vi "gyro -- async pll engine V2 owl.vi"(11 "pll engine event pair":T11) -> ()   [LabVIEW 2021]
uses:
  PID action.ctl
  pll parameters.ctl
  PID - mode.ctl
  lorentzian.ctl
  circle corners.ctl
  pll talkback data type.ctl
  server talk-to-back pair.ctl
  server talkback message type.ctl
  server talkto message type.ctl
  pid -- parameters.ctl
  owl parameters.ctl
  owl action.ctl
  owl -- send for fit action.ctl
  agregator -- action.ctl
  interpolation state - real.ctl
  launch items list.ctl
  que event bag action.ctl
  data source action.ctl
  four-corner circle transformation.ctl
  publisher action.ctl
  cursor winow.ctl
  linear interpolation - real.vi
  Q -- check range -- i -- real.vi
  linear interpolation iiii- complex.vi
  array -- sort 2D array -- Complex.vi/05c44075-957c-bc42-b6fa-2799d0bc0485.vi
  Q - not nan -- real.vi
  <vilib>/Array/Sort 2D Array - Pop Stack.vi
  <vilib>/Array/Sort 2D Array - Push Stack.vi
  array -- sort 2D array -- Complex.vi/05c44075-957c-bc42-b6fa-2799d0bc0485.vi/269d4b3b-47f5-49e3-8884-44851e4dd9d5.vi
  array -- sort 2D array -- Complex.vi/05c44075-957c-bc42-b6fa-2799d0bc0485.vi/6d99389c-673d-4efb-bf33-19b32bcf4cf8.vi
panel:
  in  "main":enum32{"Page 1", "Page 2", "Page 3"}(tab)
  in  "pll parameters":T1={"PID mode"=enum."normal", "plot time (sec)"=0.6, "dt (sec)"=0.1, "viscous time (sec)"=0.5, "dt ave time (sec)"=0.5, "PLL limit (Hz)"=5000.0} {"PLL limit (Hz)" format="%#.2f"; "dt ave time (sec)" format="%#_10f"; "viscous time (sec)" format="%#_10f"; "dt (sec)" format="%#_10f"; "plot time (sec)" format="%#_10f"}
  in  "PID parameters :{}[];'":T3={"I (sec)"=0.004634123928756344, "P (sec)"=0.008980860327047186} {"P (sec)" scale=0.01..10.0 scale format="%#_2p"; "I (sec)" scale=0.01..10.0 scale format="%#_2p"}
  out "results":T4={"ω (Hz)"=6.93618449166945e-310, "G (Hz)"=0.9683990629933289, "V (V)"=1e-323+8e-323i, "overlimit ?"=FALSE, "running lorentzian out"={"A (VHz)"=0.009142510077437082, "ω (Hz)"=0.020119879746428596, "Γ (Hz)"=0.8109571797025381, "φ (rad)"=2.007511093178386, "Q"=0.02481003960506107, "Norm  Ampl"=nan, "z∞ (V)"=0.018500144394306906-0.0037766698823995634i, "4corners"={"z (-pi/2)"=0.023947397893225086+0.01120736437940613i, "z(inf)"=0.018500144394306906-0.0037766698823995634i, "z (pi/2)"=0.0334841786561126-0.009223923381317745i, "z center"=0.028715788274668842+0.0009917204990441924i, "z(0)"=0.03893143215503078+0.005760110880487949i, "radius"=0.011273727277179521}}, "static lorentzian out"={"A (VHz)"=6.817921124952451, "ω (Hz)"=-1.0311345636926572, "Γ (Hz)"=-1.0311345636926572, "φ (rad)"=-1.0311345636926572, "Q"=-1.0311345636926572, "Norm  Ampl"=-1.0311345636926572, "z∞ (V)"=-1.0311345636926572+0.0i, "4corners"={"z (-pi/2)"=-1.0311345636926572+0.5736824521422934i, "z(inf)"=-0.5200164984937075+1.0975277942502903i, "z (pi/2)"=-1.0311345636926572+0.5736824521422934i, "z center"=-0.5136528600391839+0.580046090596817i, "z(0)"=-0.5200164984937075+1.0975277942502903i, "radius"=-1.0311345636926572}}} {"static lorentzian out"."z∞ (V)" format="%#_4p"; "static lorentzian out"."Q" format="%#_4p"; "static lorentzian out"."φ (rad)" format="%#_3p"; "static lorentzian out"."Γ (Hz)" format="%#_5p"; "static lorentzian out"."ω (Hz)" format="%#_9p"; "static lorentzian out"."A (VHz)" format="%#_3p"; "running lorentzian out"."z∞ (V)" format="%#_4p"; "running lorentzian out"."Q" format="%#_4p"; "running lorentzian out"."φ (rad)" format="%#_3p"; "running lorentzian out"."Γ (Hz)" format="%#_5p"; "running lorentzian out"."ω (Hz)" format="%#_9p"; "running lorentzian out"."A (VHz)" format="%#_3p"; "V (V)" format="%#_5p"; "G (Hz)" format="%#_5p"; "ω (Hz)" format="%#_11p"}
  out "PLL is ON ?":bool
  in  "OWL parameters":T7={"T (sec)"=3.0, "owl?"=enum."focus", "A (rad)"=0.8, "refit ?"=enum."chill"} {"T (sec)" scale=1.0..20.0; "A (rad)" scale=0.1..1.57}
  in  "publish dt (sec)":dbl=0.1 format="%#_10f"
  in  "fitter dt (sec)":dbl=0.1 format="%#_10f"
  in  "Do reset frequency -- PID action":T10=enum."reset frequency"
  in  "Do reset frequency source":dbl=15.0 format="%#_10f"
  out "zi freq temporary":dbl=46378.93366130424 format="%#.2f"
  out "DO reset freq !":bool
  in  "lorentzian":T5={"A (VHz)"=0.009142510077437082, "ω (Hz)"=0.020119879746428596, "Γ (Hz)"=0.8109571797025381, "φ (rad)"=2.007511093178386, "Q"=0.02481003960506107, "Norm  Ampl"=nan, "z∞ (V)"=0.018500144394306906-0.0037766698823995634i, "4corners"={"z (-pi/2)"=0.023947397893225086+0.01120736437940613i, "z(inf)"=0.018500144394306906-0.0037766698823995634i, "z (pi/2)"=0.0334841786561126-0.009223923381317745i, "z center"=0.028715788274668842+0.0009917204990441924i, "z(0)"=0.03893143215503078+0.005760110880487949i, "radius"=0.011273727277179521}} {"z∞ (V)" format="%#_4p"; "Q" format="%#_4p"; "φ (rad)" format="%#_3p"; "Γ (Hz)" format="%#_5p"; "ω (Hz)" format="%#_9p"; "A (VHz)" format="%#_3p"}
  out "PLL loop Stoped?":bool=TRUE
  out "publish loop Stoped?":bool=TRUE
  out "fitter loop Stoped?":bool=TRUE
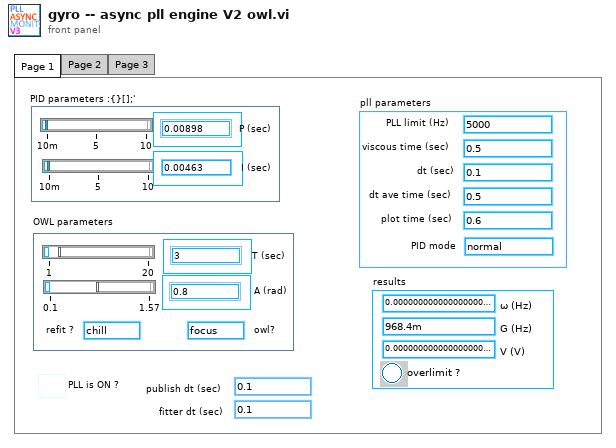
[diagram p1: front panel]
types:
  T1 = typedef "pll parameters.ctl" = cluster{"PID mode":T2, "plot time (sec)":dbl, "dt (sec)":dbl, "viscous time (sec)":dbl, "dt ave time (sec)":dbl, "PLL limit (Hz)":dbl}
  T2 = typedef "PID - mode.ctl" = enum16{"normal", "heat"}
  T3 = typedef "pid -- parameters.ctl" = cluster{"I (sec)":dbl, "P (sec)":dbl}
  T4 = typedef "pll talkback data type.ctl" = cluster{"ω (Hz)":dbl, "G (Hz)":dbl, "V (V)":cdb, "overlimit ?":bool, "running lorentzian out":T5, "static lorentzian out":T5}
  T5 = typedef "lorentzian.ctl" = cluster{"A (VHz)":dbl, "ω (Hz)":dbl, "Γ (Hz)":dbl, "φ (rad)":dbl, "Q":dbl, "Norm  Ampl":dbl, "z∞ (V)":cdb, "4corners":T6}
  T6 = typedef "circle corners.ctl" = cluster{"z (-pi/2)":cdb, "z(inf)":cdb, "z (pi/2)":cdb, "z center":cdb, "z(0)":cdb, "radius":dbl}
  T7 = typedef "owl parameters.ctl" = cluster{"T (sec)":dbl, "owl?":T8, "A (rad)":dbl, "refit ?":T9}
  T8 = typedef "owl action.ctl" = enum16{"owl", "focus"}
  T9 = typedef "owl -- send for fit action.ctl" = enum16{"refit", "chill"}
  T10 = typedef "PID action.ctl" = enum16{"append", "empty!", "reset frequency", "reset from num", "overlimit"}
  T11 = typedef "server talk-to-back pair.ctl" = cluster{"talkback event":refnum<user-event>, "talkto event":refnum<user-event>}
  T12 = typedef "launch items list.ctl" = enum16{"source", "pll engine", "pll monitor", "sweeper engine", "sweeper monitor", "fitter"}
  T13 = typedef "que event bag action.ctl" = enum16{"check", "add", "init", "keys", "values"}
  T14 = typedef "interpolation state - real.ctl" = cluster{"Array ":dbl[], "actual size":i32, "requested size":i32}
  T15 = typedef "agregator -- action.ctl" = enum16{"append", "interpolate", "empty!", "force", "init", "scale", "read last"}
  T16 = typedef "publisher action.ctl" = enum16{"set", "get", "init", "check"}
  T17 = typedef "server talkto message type.ctl" = cluster{"message":enum16{"stop", "start", "update pars", "update request", "new", "launch", "exit", "get", "reset", "pause", "unpause"}}
  T18 = typedef "data source action.ctl" = enum16{"set", "get", "init", "set-and-get", "init source"}
  T19 = typedef "four-corner circle transformation.ctl" = enum16{"z(c) z(inf)", "z(c) z(zero)", "fix phase", "calculate lorentzian", "z(0) z(+-pi/2)", "shift to zcenter", "to  canonical", "get canonical phase", "get4corners", "update lorentzian -- from z0", "fake gamma normal", "fake gamma heat", "calculate complex slope", "get f0 given f and phi"}
  T20 = typedef "cursor winow.ctl" = cluster{"left":dbl, "right ":dbl, "center":dbl, "window":dbl, "cursors":i32[], "relative":i32, "absolute":i32, "fixed vertical offset":dbl, "vertical offset":dbl, "skew":dbl, "default window frac":dbl, "kind":enum16{"symmetric", "skewed", "fancy"}, "skew.left":dbl, "skew.right":dbl, "Plot ref":refnum<vi>, "wing order":enum16{"forw", "back"}}
  T21 = typedef "PLL data source.ctl" = enum16{"meta", "MFLI", "SRS865A", "arydh"}
  T22 = typedef "interpolation state - complex.ctl" = cluster{"requested size":i32, "Array":cdb[], "actual number of elements":i32}
  T23 = typedef "server talkback message type.ctl" = cluster{"message":enum16{"new", "void"}}
  T24 = typedef "eventvkey.ctl" = enum16{"ASCII", "Enter", "Return", "Shift", "Ctrl", "Alt", "Cmd", "Opt", "Caps", "NumLock", "Clear", "Break", "Up", "Down", "Left", "Right", "Insert", "Delete", "Home", "End", "PageUp", "PageDown", "Escape", "Help", "Pause", "ScrollLock", "F1", "F2", "F3", "F4", "F5", "F6", "F7", "F8", "F9", "F10", "F11", "F12", "F13", "F14", "F15", "F16", "F17", "F18", "F19", "F20", "F21", "F22", "F23", "F24", "Play", "VolumeUp", "VolumeDown", "Mute", "Two Byte Char"}
  T25 = enum16{"stop", "start", "update pars", "update request", "new", "launch", "exit", "get", "reset", "pause", "unpause"}
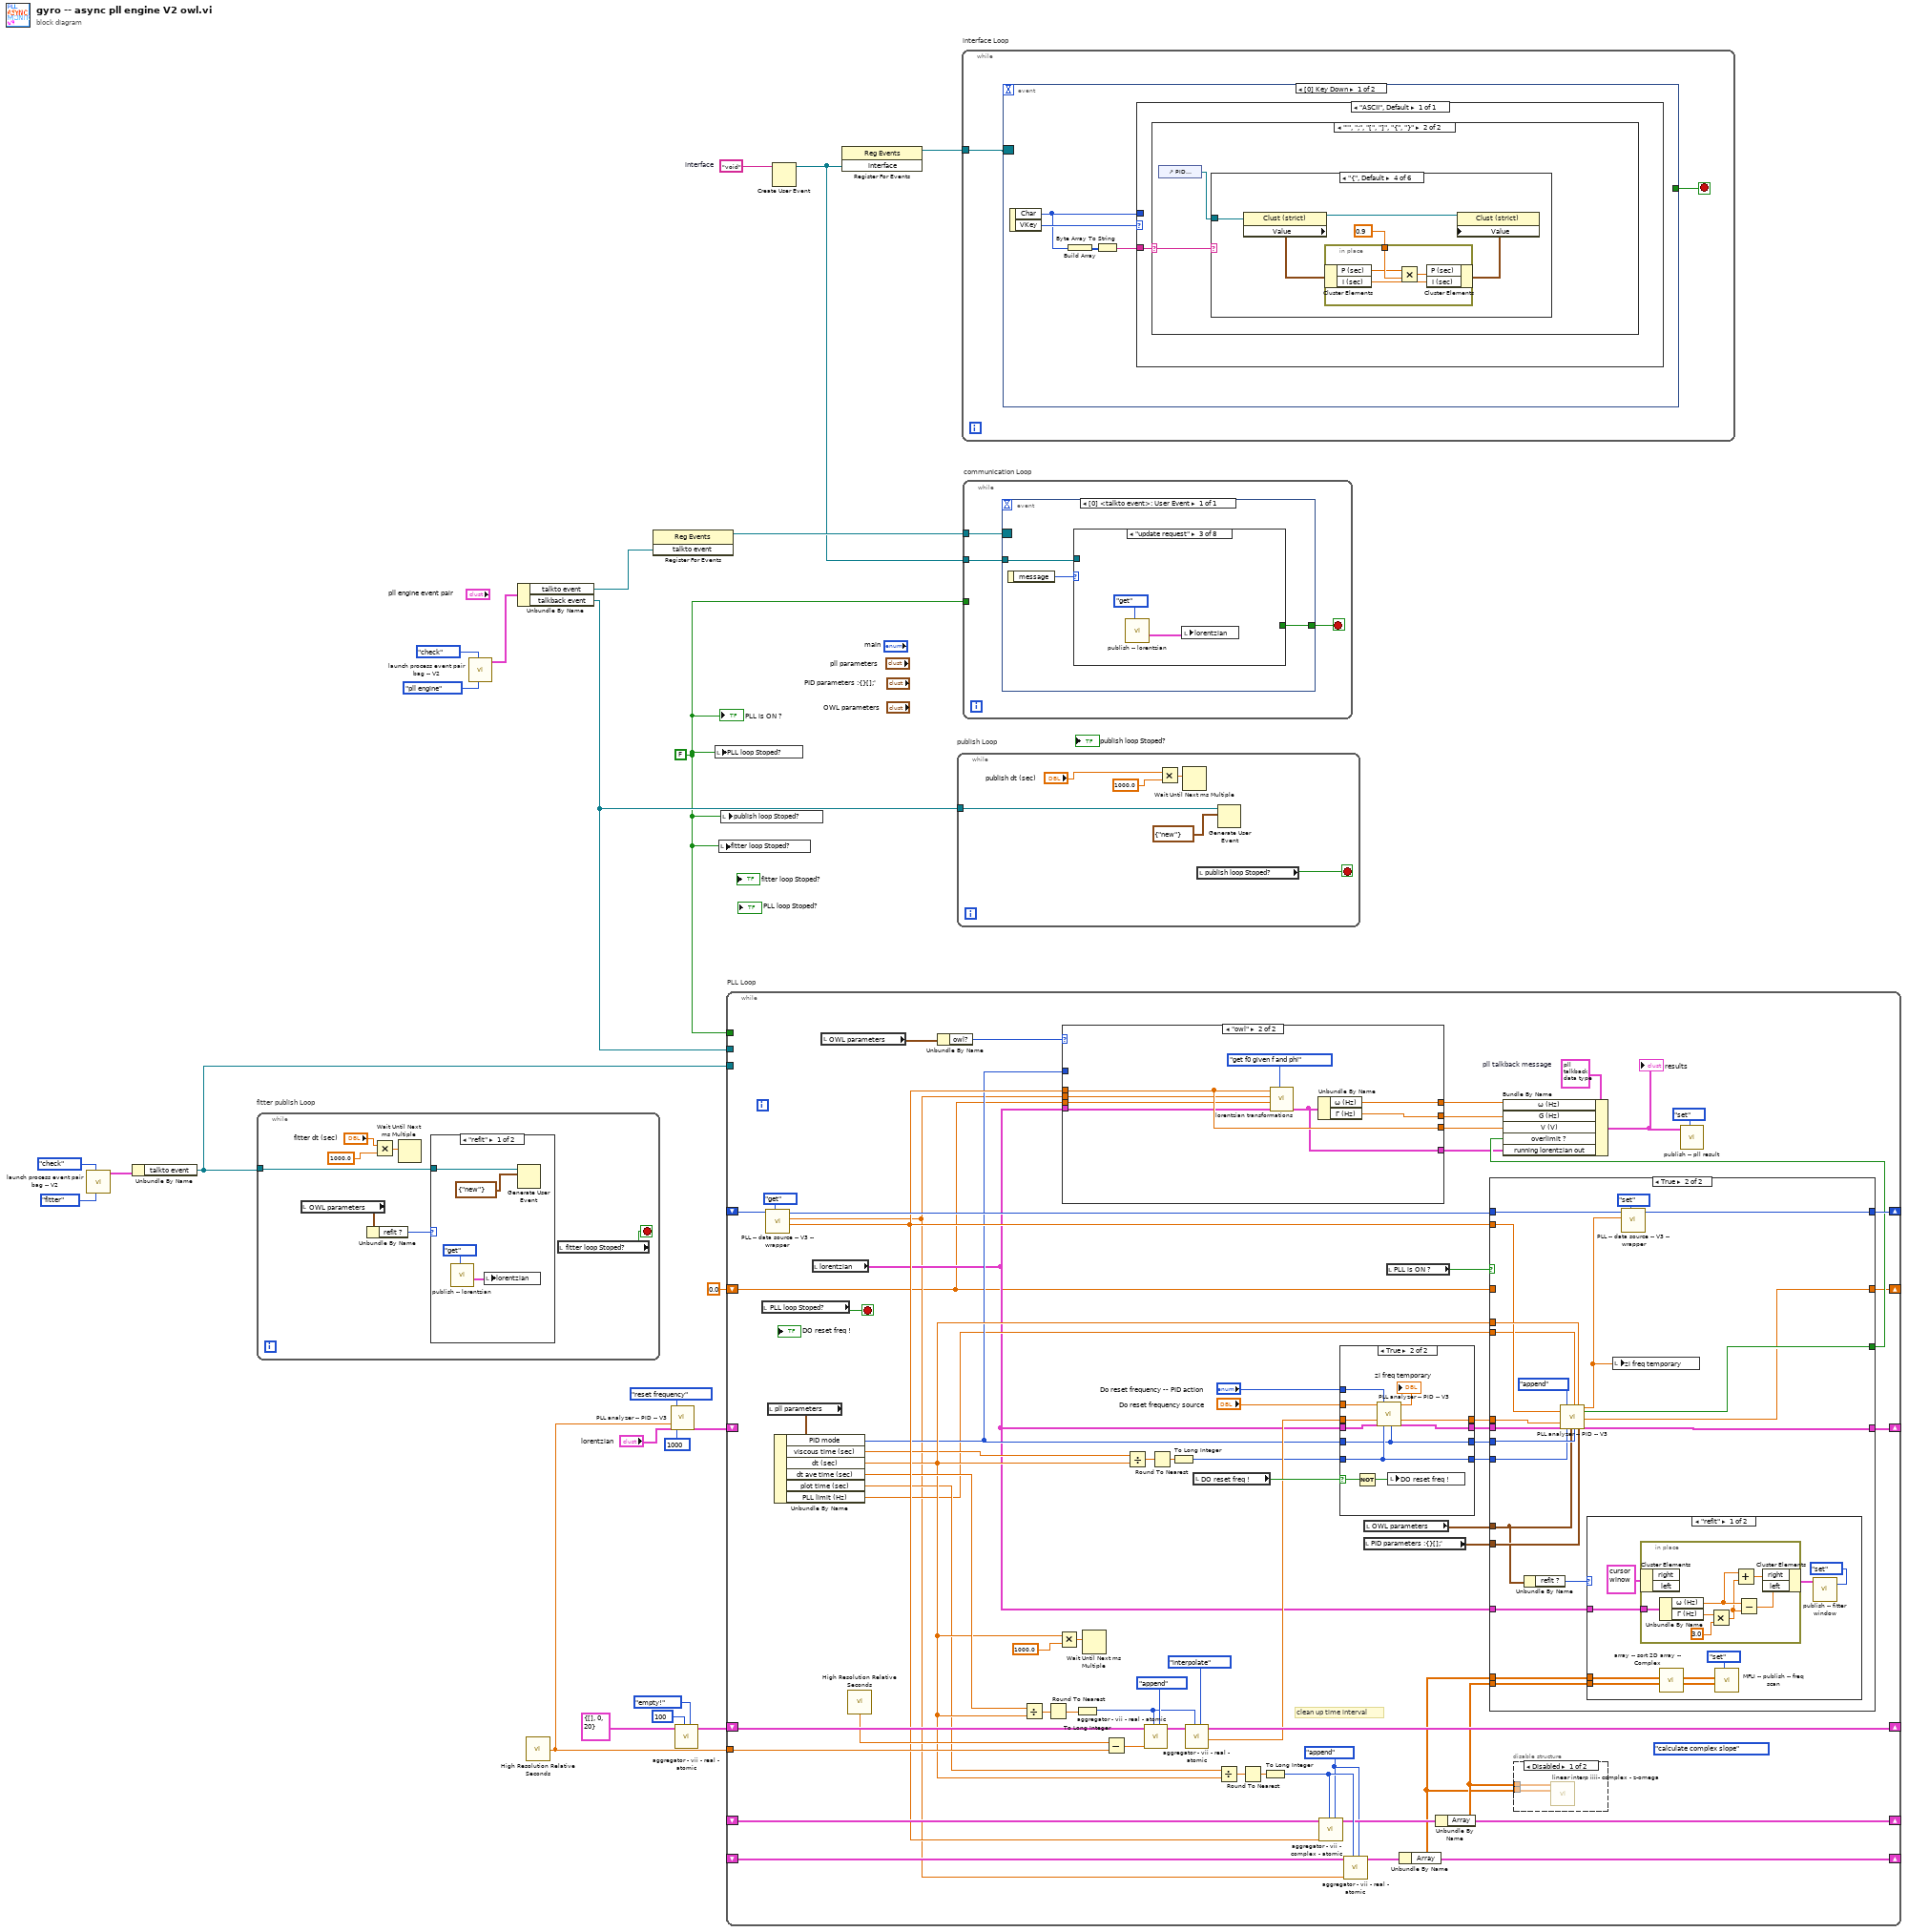
[diagram p0: block diagram]
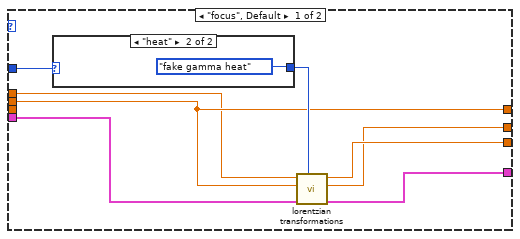
[diagram p3: hidden frame]
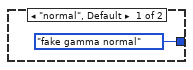
[diagram p4: hidden frame]
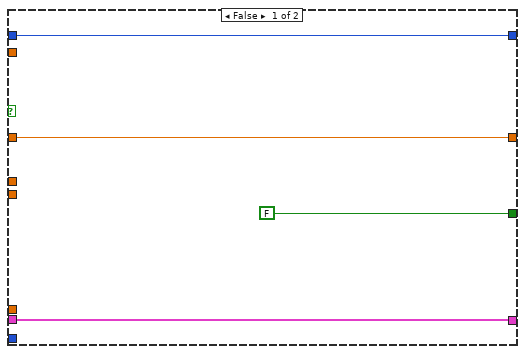
[diagram p6: hidden frame]
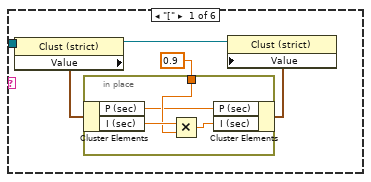
[diagram p10: hidden frame]
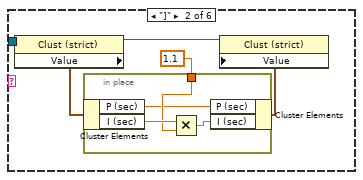
[diagram p11: hidden frame]
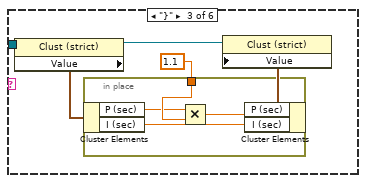
[diagram p12: hidden frame]
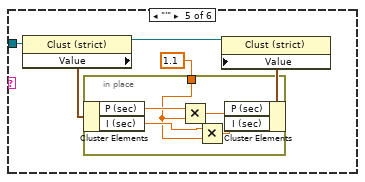
[diagram p13: hidden frame]
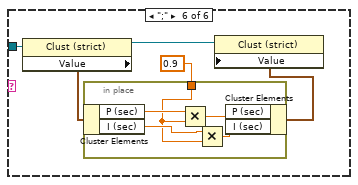
[diagram p14: hidden frame]
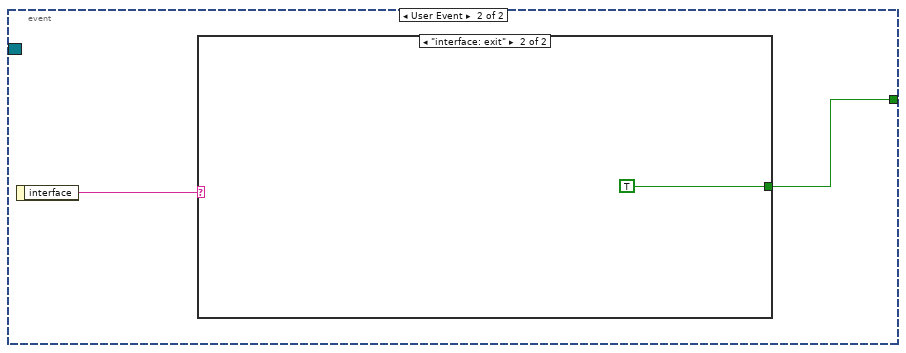
[diagram p15: hidden frame]
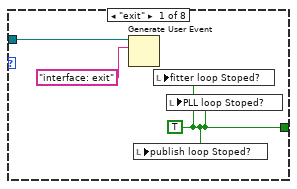
[diagram p17: hidden frame]
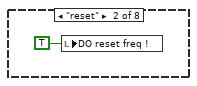
[diagram p18: hidden frame]
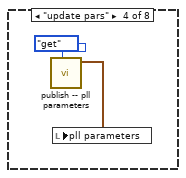
[diagram p19: hidden frame]
diagram:
  w13 = "void"  # interface
  w3 = FALSE ("Stop")
  n1 = call "launch process event pair bag -- V2.vi"("launch item"=launch_items_list."fitter" ("launch items"), "bag action"=que_event_bag_action."check") -> ("event pair OUT"=w4:T11)  [unwired: 7 in, 2 out]
  n2 = Unbundle By Name(w4) -> ("talkto event"=w2:refnum<user-event>)
  n3 = while "fitter publish Loop" {
    tunnel: w2 -> [w31]
    stop <- w30 stop-if-true
    n4 = local read "OWL parameters"() -> (w26:T7)
    n5 = Unbundle By Name(w26) -> ("refit ?"=w25:T9)
    n6 = Multiply(x="fitter dt (sec)", y=1000.0) -> (x*y=w27:dbl)
    n7 = Wait Until Next ms Multiple(millisecond multiple=w27) -> ()  [unwired: 1 out]
    n8 = case shown="\"refit\"" w25 {
      tunnel: w31 -> [w35 _]
      frame "refit" {
        n9 = call "publish -- lorentzian.vi"("publisher action"=publisher_action."get") -> ("lorentzian OUT"=w32:T5)  [unwired: 10 in]
        n10 = local write "lorentzian"(w32) -> ()
        n11 = Generate User Event(user event=w35, event data cluster=T17 {"message"=enum."new"} ("event data")) -> ()  [unwired: 2 in, 2 out]
      }
      frame "chill", Default {
      }
    }
    n12 = local read "fitter loop Stoped?"() -> (w30:bool)
  }
  n13 = call "launch process event pair bag -- V2.vi"("launch item"=launch_items_list."pll engine" ("launch items"), "bag action"=que_event_bag_action."check") -> ("event pair OUT"=w7:T11)  [unwired: 7 in, 2 out]
  n14 = Unbundle By Name(w7) -> ("talkto event"=w23:refnum<user-event>, "talkback event"=w10:refnum<user-event>)
  n15 = call <vilib>:"High Resolution Relative Seconds.vi"() -> ("relative seconds"=w15:dbl)
  n16 = register-events(w23) -> (reference out=w24:refnum<event-registration>)  [unwired: 2 in, 1 out]
  n17 = call "PLL analyzer -- PID -- V3.vi"("time in (sec)"=w15, "lorentzian IN"="lorentzian", "PID action"=PID_action."reset frequency", "requested size"=1000) -> ("lorentzian  OUT"=w18:T5)  [unwired: 11 in, 4 out]
  n18 = call "aggregator - vii - real - atomic.vi"("aggregator action"=agregator_--_action."empty!", "requested size"=100, "state IN"=T14 {"Array "=[], "actual size"=0, "requested size"=20}) -> ("state OUT"=w21:T14)  [unwired: 5 in, 3 out]
  n19 = local write "PLL loop Stoped?"(w3) -> ()
  n20 = local write "fitter loop Stoped?"(w3) -> ()
  n21 = local write "publish loop Stoped?"(w3) -> ()
  n22 = while "PLL Loop" {
    tunnel: w15 -> [w100]
    shift-right: [w98] -> _
    shift-left: w18 -> [_]
    shift-right: [w66] -> _
    shift-left: _ -> [w97]
    shift-right: [w95] -> _
    shift-left: _ -> [w96]
    shift-right: [w90] -> _
    shift-left: w21 -> [w93]
    shift-right: [w85] -> _
    shift-left: _ -> [w81]
    tunnel: w10 -> [_]
    tunnel: w3 -> [_]
    tunnel: w2 -> [_]
    shift-right: [w37] -> _
    shift-left: 0.0 ("phase OUT (rad)") -> [w36]
    stop <- w51 stop-if-true
    w62 = T4 {"ω (Hz)"=0.0, "G (Hz)"=0.0, "V (V)"=0.0+0.0i, "overlimit ?"=FALSE, "running lorentzian out"={"A (VHz)"=-1.0311345636926572, "ω (Hz)"=-1.0311345636926572, "Γ (Hz)"=-1.0311345636926572, "φ (rad)"=-1.0311345636926572, "Q"=-1.0311345636926572, "Norm  Ampl"=-1.0311345636926572, "z∞ (V)"=-1.0311345636926572+0.0i, "4corners"={"z (-pi/2)"=-1.0311345636926572+0.5736824521422934i, "z(inf)"=-0.5200164984937075+1.0975277942502903i, "z (pi/2)"=-1.0311345636926572+0.5736824521422934i, "z center"=-0.5136528600391839+0.580046090596817i, "z(0)"=-0.5200164984937075+1.0975277942502903i, "radius"=-1.0311345636926572}}, "static lorentzian out"={"A (VHz)"=6.817921124952451, "ω (Hz)"=-1.0311345636926572, "Γ (Hz)"=-1.0311345636926572, "φ (rad)"=-1.0311345636926572, "Q"=-1.0311345636926572, "Norm  Ampl"=-1.0311345636926572, "z∞ (V)"=-1.0311345636926572+0.0i, "4corners"={"z (-pi/2)"=-1.0311345636926572+0.5736824521422934i, "z(inf)"=-0.5200164984937075+1.0975277942502903i, "z (pi/2)"=-1.0311345636926572+0.5736824521422934i, "z center"=-0.5136528600391839+0.580046090596817i, "z(0)"=-0.5200164984937075+1.0975277942502903i, "radius"=-1.0311345636926572}}}  # pll talkback message
    (unwired) four-corner_circle_transformation."calculate complex slope" ("4 corner circle transformation")
    w48 = agregator_--_action."append" ("aggregator action")
    # "clean up time interval"
    n23 = local read "PLL loop Stoped?"() -> (w51:bool)
    n24 = call "PLL -- data source -- V3 -- wrapper.vi"("data source action"=data_source_action."get", "PLL data source"=w81) -> ("z out (V)"=w63:cdb, "Freq out (Hz)"=w43:dbl, "PLL data source OUT"=w83:T21)  [unwired: 7 in]
    n25 = local read "pll parameters"() -> (w57:T1)
    n26 = Unbundle By Name(w57) -> ("PID mode"=w58:T2, "viscous time (sec)"=w59:dbl, "dt (sec)"=w60:dbl, "dt ave time (sec)"=w61:dbl, "plot time (sec)"=w56:dbl, "PLL limit (Hz)"=w54:dbl)
    n27 = local read "lorentzian"() -> (w44:T5)
    n28 = local read "OWL parameters"() -> (w39:T7)
    n29 = call <vilib>:"High Resolution Relative Seconds.vi"() -> ("relative seconds"=w84:dbl)
    n30 = Unbundle By Name(w39) -> ("owl?"=w40:T8)
    n31 = Divide(x=w61, y=w60) -> (x/y=w74:dbl)
    n32 = Round To Nearest(number=w74) -> (nearest integer value=w73:dbl)
    n33 = Multiply(x=w60, y=1000.0) -> (x*y=w88:dbl)
    n34 = case shown="\"owl\"" w40 {
      tunnel: [w101 w114] -> w64
      tunnel: w63 -> [w103 w116]
      tunnel: w58 -> [w105 _]
      tunnel: w44 -> [w102 w112]
      tunnel: w43 -> [w104 w113]
      tunnel: [w104 w111] -> w42
      tunnel: [w103 w116] -> w41
      tunnel: [w102 w110] -> w38
      tunnel: w36 -> [_ w109]
      frame "focus", Default {
        n35 = case shown="\"heat\"" w105 {
          tunnel: [four-corner_circle_transformation."fake gamma normal" ("4 corner circle transformation") four-corner_circle_transformation."fake gamma heat" ("4 corner circle transformation")] -> w106
          frame "normal", Default {
          }
          frame "heat" {
          }
        }
        n36 = call "lorentzian transformations.vi"("4 corner circle transformation"=w106, "lorentzian in"=w102, "freq in"=w104, "voltage in"=w103) -> ("gamma OUT"=w101:dbl)  [unwired: 4 in, 3 out]
      }
      frame "owl" {
        n37 = call "lorentzian transformations.vi"("4 corner circle transformation"=four-corner_circle_transformation."get f0 given f and phi", "lorentzian in"=w112, "phase in (rad)"=w109, "freq in"=w113, "voltage in"=w116) -> ("lorentzian out"=w110:T5)  [unwired: 3 in, 3 out]
        n38 = Unbundle By Name(w110) -> ("ω (Hz)"=w111:dbl, "Γ (Hz)"=w114:dbl)
      }
    }
    n39 = To Long Integer(number=w73) -> (32bit integer=w72:i32)
    n40 = Wait Until Next ms Multiple(millisecond multiple=w88) -> ()  [unwired: 1 out]
    n41 = Subtract(x=w84, y=w100) -> (x-y=w92:dbl)
    n42 = Divide(x=w59, y=w60) -> (x/y=w77:dbl)
    n43 = call "aggregator - vii - real - atomic.vi"("aggregator action"=agregator_--_action."append", "requested size"=w72, "number"=w92, "state IN"=w93) -> ("state OUT"=w91:T14)  [unwired: 4 in, 3 out]
    n44 = Round To Nearest(number=w77) -> (nearest integer value=w76:dbl)
    n45 = To Long Integer(number=w76) -> (32bit integer=w75:i32)
    n46 = call "aggregator - vii - real - atomic.vi"("aggregator action"=agregator_--_action."interpolate", "requested size"=w72, "state IN"=w91) -> ("interp average"=w79:dbl, "state OUT"=w90:T14)  [unwired: 5 in, 2 out]
    n47 = local read "DO reset freq !"() -> (w87:bool)
    n48 = Divide(x=w56, y=w60) -> (x/y=w70:dbl)
    n49 = Round To Nearest(number=w70) -> (nearest integer value=w69:dbl)
    n50 = To Long Integer(number=w69) -> (32bit integer=w68:i32)
    n51 = call "aggregator - vii - complex - atomic.vi"("aggregator action"=w48, "requested size"=w68, "number"=w63, "state IN"=w97) -> ("state OUT"=w66:T22)  [unwired: 4 in, 3 out]
    n52 = case shown="True" w87 {
      selector: w87 -> [_ w172]
      tunnel: w44 -> [w163 w174]
      tunnel: [w163 w173] -> w86
      tunnel: w75 -> [w162 w169]
      tunnel: [w162 w169] -> w80
      tunnel: w79 -> [w161 w168]
      tunnel: "Do reset frequency -- PID action" -> [_ w167]
      tunnel: "Do reset frequency source" -> [_ w166]
      tunnel: [w161 w165] -> w71
      tunnel: w58 -> [w160 w164]
      tunnel: [w160 w164] -> w67
      frame False {
      }
      frame True {
        n53 = Not(x=w172) -> (.not. x?=w171:bool)
        n54 = call "PLL analyzer -- PID -- V3.vi"("frequency IN (Hz)"=w166, "time in (sec)"=w168, "lorentzian IN"=w174, "PID action"=w167, "requested size"=w169, "PID mode"=w164) -> ("frequency OUT (Hz)"=→"zi freq temporary":dbl, "time out (sec)"=w165:dbl, "lorentzian  OUT"=w173:T5)  [unwired: 9 in, 2 out]
        n55 = local write "DO reset freq !"(w171) -> ()
      }
    }
    n56 = call "aggregator - vii - real - atomic.vi"("aggregator action"=w48, "requested size"=w68, "number"=w43, "state IN"=w96) -> ("state OUT"=w95:T14)  [unwired: 4 in, 3 out]
    n57 = local read "PID parameters :{}[];'"() -> (w49:T3)
    n58 = local read "OWL parameters"() -> (w47:T7)
    n59 = local read "PLL is ON ?"() -> (w50:bool)
    n60 = Unbundle By Name(w95) -> ("Array"=w45:dbl[])
    n61 = Unbundle By Name(w66) -> ("Array"=w46:cdb[])
    n62 = case shown="True" w50 {
      tunnel: [w122 w143] -> w98
      tunnel: w80 -> [_ w134]
      tunnel: w63 -> [_ w133]
      tunnel: w71 -> [_ w138]
      tunnel: w86 -> [w122 w135]
      tunnel: [w121 w141] -> w85
      tunnel: w83 -> [w121 w139]
      tunnel: w60 -> [_ w137]
      tunnel: w67 -> [_ w136]
      tunnel: w49 -> [_ w132]
      tunnel: [FALSE w131] -> w55
      tunnel: w54 -> [_ w130]
      tunnel: w47 -> [_ w127]
      tunnel: w46 -> [_ w129]
      tunnel: w45 -> [_ w128]
      tunnel: w44 -> [_ w125]
      tunnel: [w119 w123] -> w37
      tunnel: w36 -> [w119 _]
      frame False {
      }
      frame True {
        n63 = Unbundle By Name(w127) -> ("refit ?"=w126:T9)
        n64 = call "PLL analyzer -- PID -- V3.vi"("voltage IN (V)"=w133, "time in (sec)"=w138, "lorentzian IN"=w135, "PID action"=PID_action."append", "requested size"=w134, "OWL parameters"=w127, "PLL limits (Hz)"=w130, "PID mode"=w136, "dt (sec)"=w137, "PID parameters"=w132) -> ("frequency OUT (Hz)"=w124:dbl, "overlimit ?"=w131:bool, "phase OUT (rad)"=w123:dbl, "lorentzian  OUT"=w143:T5)  [unwired: 5 in, 1 out]
        n65 = case shown="\"refit\"" w126 {
          tunnel: w129 -> [w145 _]
          tunnel: w128 -> [w147 _]
          tunnel: w125 -> [w149 _]
          frame "refit" {
            n66 = in-place {
              in-place-border: w149 -> [w159]
              n67 = in-place-cluster #1(T20 {"left"=-0.35260838541595674, "right "=17.234446484426172, "center"=-8.969831627629043, "window"=8.26461485679713, "cursors"=[], "relative"=0, "absolute"=0, "fixed vertical offset"=2421.6740576496672, "vertical offset"=2421.6740576496672, "skew"=2421.6740576496672, "default window frac"=2421.6740576496672, "kind"=enum."skewed", "skew.left"=2421.6740576496672, "skew.right"=2421.6740576496672, "Plot ref"=refnum, "wing order"=enum."back"} ("win OUT")) -> ()  [unwired: 2 out]
              n68 = Unbundle By Name(w159) -> ("ω (Hz)"=w156:dbl, "Γ (Hz)"=w158:dbl)
              n69 = Multiply(x=w158, y=3.0) -> (x*y=w155:dbl)
              n70 = Add(x=w156, y=w155) -> (x+y=w154:dbl)
              n71 = Subtract(x=w156, y=w155) -> (x-y=w153:dbl)
              n72 = in-place-cluster #1("right"=w154, "left"=w153) -> (w150:T20)
            }
            n73 = call "array -- sort 2D array -- Complex.vi"("z In"=w145, "freq IN"=w147) -> ("z out"=w144:cdb[], "freq out"=w146:dbl[])  [unwired: 8 in]
            n74 = call "MFLI -- publish -- freq scan.vi"("publisher action"=publisher_action."set", "Voltage IN (V)"=w144, "Freq IN (Hz)"=w146) -> ()  [unwired: 7 in, 2 out]
            n75 = call "publish -- fitter window.vi"("publisher action"=publisher_action."set", "win IN"=w150) -> ()  [unwired: 9 in, 1 out]
          }
          frame "chill", Default {
          }
        }
        n76 = local write "zi freq temporary"(w124) -> ()
        n77 = call "PLL -- data source -- V3 -- wrapper.vi"("data source action"=data_source_action."set", "Freq in (Hz)"=w124, "PLL data source"=w139) -> ("PLL data source OUT"=w141:T21)  [unwired: 6 in, 2 out]
      }
    }
    n78 = Bundle By Name(cluster=w62, "ω (Hz)"=w42, "G (Hz)"=w64, "V (V)"=w41, "overlimit ?"=w55, "running lorentzian out"=w38) -> (w53:T4)
    "results" <- w53
    n79 = disable-structure shown="Disabled" {
      disable-tunnel: w46 -> [w118 _]
      disable-tunnel: w45 -> [w117 _]
      frame Disabled {
        n80 = call "linear interp iiii- complex - z-omega.vi"("z"=w118, "omega"=w117) -> ()  [unwired: 5 in, 9 out]
      }
      frame Enabled {
      }
    }
    n81 = call "publish -- pll result.vi"("publisher action"=publisher_action."set", "pll result IN"=w53) -> ()  [unwired: 9 in, 1 out]
  }
  n82 = Create User Event(user event datatype=w13) -> (user event=w11:refnum<user-event>)  [unwired: 1 in, 1 out]
  n83 = register-events(w11) -> (reference out=w12:refnum<event-registration>)  [unwired: 2 in, 1 out]
  n84 = while "publish Loop" {
    tunnel: w10 -> [w179]
    stop <- w178 stop-if-true
    n85 = Multiply(x="publish dt (sec)", y=1000.0) -> (x*y=w175:dbl)
    n86 = Wait Until Next ms Multiple(millisecond multiple=w175) -> ()  [unwired: 1 out]
    n87 = local read "publish loop Stoped?"() -> (w178:bool)
    n88 = Generate User Event(user event=w179, event data cluster=T23 {"message"=enum."new"} ("event data")) -> ()  [unwired: 2 in, 2 out]
  }
  n89 = while "interface Loop" {
    tunnel: w12 -> [w182]
    stop <- w181 stop-if-true
    n90 = event shown="[0] Key Down" {
      selector: w182 -> [_ _]
      dyn-events: _ -> [_ _]
      timeout: _ -> [_ _]
      tunnel: [_ w246] -> w181
      event Key Down {
        n91 = event-data() -> ("Char"=w184:i16, "VKey"=w186:T24)  [unwired: 1 in]
        n92 = Build Array(w184) -> (w185:i16[])
        n93 = Byte Array To String(unsigned byte array=w185) -> (string=w183:string)
        n94 = case shown="\"ASCII\", Default" w186 {
          tunnel: w184 -> [_]
          tunnel: w183 -> [w187]
          frame "ASCII", Default {
            n95 = case shown="\"'\", \";\", \"[\", \"]\", \"{\", \"}\"" w187 {
              selector: w187 -> [_ w189]
              frame "0", Default {
              }
              frame "'", ";", "[", "]", "{", "}" {
                n96 = control-ref of="PID parameters :{}[];'"() -> (w188:refnum<vi>)
                n97 = case shown="\"{\", Default" w189 {
                  tunnel: w188 -> [w194 w203 w212 w221 w230 w240]
                  frame "[" {
                    n98 = property class="Clust (strict)"(reference=w194) -> (reference out=w193:refnum<vi>, "Value"=w192:T3)  [unwired: 1 in, 1 out]
                    n99 = in-place {
                      in-place-border: 0.9 -> [w197]
                      n100 = in-place-cluster #2(w192) -> ("P (sec)"=w195:dbl, "I (sec)"=w198:dbl)
                      n101 = Multiply(x=w198, y=w197) -> (x*y=w196:dbl)
                      n102 = in-place-cluster #2("P (sec)"=w195, "I (sec)"=w196) -> (w191:T3)
                    }
                    n103 = property class="Clust (strict)"(reference=w193, "Value"=w191) -> ()  [unwired: 1 in, 2 out]
                  }
                  frame "]" {
                    n104 = property class="Clust (strict)"(reference=w203) -> (reference out=w202:refnum<vi>, "Value"=w201:T3)  [unwired: 1 in, 1 out]
                    n105 = in-place {
                      in-place-border: 1.1 -> [w206]
                      n106 = in-place-cluster #3(w201) -> ("P (sec)"=w204:dbl, "I (sec)"=w207:dbl)
                      n107 = Multiply(x=w207, y=w206) -> (x*y=w205:dbl)
                      n108 = in-place-cluster #3("P (sec)"=w204, "I (sec)"=w205) -> (w200:T3)
                    }
                    n109 = property class="Clust (strict)"(reference=w202, "Value"=w200) -> ()  [unwired: 1 in, 2 out]
                  }
                  frame "}" {
                    n110 = property class="Clust (strict)"(reference=w212) -> (reference out=w211:refnum<vi>, "Value"=w210:T3)  [unwired: 1 in, 1 out]
                    n111 = in-place {
                      in-place-border: 1.1 -> [w216]
                      n112 = in-place-cluster #4(w210) -> ("P (sec)"=w215:dbl, "I (sec)"=w213:dbl)
                      n113 = Multiply(x=w215, y=w216) -> (x*y=w214:dbl)
                      n114 = in-place-cluster #4("P (sec)"=w214, "I (sec)"=w213) -> (w209:T3)
                    }
                    n115 = property class="Clust (strict)"(reference=w211, "Value"=w209) -> ()  [unwired: 1 in, 2 out]
                  }
                  frame "{", Default {
                    n116 = property class="Clust (strict)"(reference=w221) -> (reference out=w220:refnum<vi>, "Value"=w219:T3)  [unwired: 1 in, 1 out]
                    n117 = in-place {
                      in-place-border: 0.9 -> [w225]
                      n118 = in-place-cluster #5(w219) -> ("P (sec)"=w224:dbl, "I (sec)"=w222:dbl)
                      n119 = Multiply(x=w224, y=w225) -> (x*y=w223:dbl)
                      n120 = in-place-cluster #5("P (sec)"=w223, "I (sec)"=w222) -> (w218:T3)
                    }
                    n121 = property class="Clust (strict)"(reference=w220, "Value"=w218) -> ()  [unwired: 1 in, 2 out]
                  }
                  frame "'" {
                    n122 = property class="Clust (strict)"(reference=w230) -> (reference out=w229:refnum<vi>, "Value"=w228:T3)  [unwired: 1 in, 1 out]
                    n123 = in-place {
                      in-place-border: 1.1 -> [w231]
                      n124 = in-place-cluster #6(w228) -> ("P (sec)"=w235:dbl, "I (sec)"=w233:dbl)
                      n125 = Multiply(x=w235, y=w231) -> (x*y=w234:dbl)
                      n126 = Multiply(x=w233, y=w231) -> (x*y=w232:dbl)
                      n127 = in-place-cluster #6("P (sec)"=w234, "I (sec)"=w232) -> (w227:T3)
                    }
                    n128 = property class="Clust (strict)"(reference=w229, "Value"=w227) -> ()  [unwired: 1 in, 2 out]
                  }
                  frame ";" {
                    n129 = property class="Clust (strict)"(reference=w240) -> (reference out=w239:refnum<vi>, "Value"=w238:T3)  [unwired: 1 in, 1 out]
                    n130 = in-place {
                      in-place-border: 0.9 -> [w241]
                      n131 = in-place-cluster #7(w238) -> ("P (sec)"=w245:dbl, "I (sec)"=w243:dbl)
                      n132 = Multiply(x=w245, y=w241) -> (x*y=w244:dbl)
                      n133 = Multiply(x=w243, y=w241) -> (x*y=w242:dbl)
                      n134 = in-place-cluster #7("P (sec)"=w244, "I (sec)"=w242) -> (w237:T3)
                    }
                    n135 = property class="Clust (strict)"(reference=w239, "Value"=w237) -> ()  [unwired: 1 in, 2 out]
                  }
                }
              }
            }
          }
        }
      }
      event User Event {
        n136 = event-data() -> ("interface"=w247:string)  [unwired: 1 in]
        n137 = case shown="\"interface: exit\"" w247 {
          tunnel: [_ TRUE] -> w246
          frame "False", Default {
          }
          frame "interface: exit" {
          }
        }
      }
    }
  }
  n138 = while "communication Loop" {
    tunnel: w24 -> [w251]
    tunnel: w3 -> [_]
    tunnel: w11 -> [w249]
    stop <- w250 stop-if-true
    n139 = event shown="[0] <talkto event>: User Event" {
      selector: w251 -> [_]
      dyn-events: _ -> [_]
      timeout: _ -> [_]
      tunnel: [w253] -> w250
      tunnel: w249 -> [w252]
      event User Event {
        n140 = event-data() -> ("message"=w254:T25)  [unwired: 1 in]
        n141 = case shown="\"update request\"" w254 {
          tunnel: [w255 _ _ _ _ _ _ _] -> w253
          tunnel: w252 -> [w257 _ _ _ _ _ _ _]
          frame "exit" {
            w255 = TRUE
            n142 = Generate User Event(user event=w257, event data cluster="interface: exit" ("event data")) -> ()  [unwired: 2 in, 2 out]
            n143 = local write "publish loop Stoped?"(w255) -> ()
            n144 = local write "fitter loop Stoped?"(w255) -> ()
            n145 = local write "PLL loop Stoped?"(w255) -> ()
          }
          frame "reset" {
            n146 = local write "DO reset freq !"(TRUE) -> ()
          }
          frame "update request" {
            n147 = call "publish -- lorentzian.vi"("publisher action"=publisher_action."get") -> ("lorentzian OUT"=w259:T5)  [unwired: 10 in]
            n148 = local write "lorentzian"(w259) -> ()
          }
          frame "update pars" {
            n149 = call "publish -- pll parameters.vi"("publisher action"=publisher_action."get") -> ("pll parameters OUT"=w261:T1)  [unwired: 10 in]
            n150 = local write "pll parameters"(w261) -> ()
          }
          frame "start", Default {
          }
          frame "stop" {
          }
          frame "pause" {
            n151 = local write "PLL is ON ?"(FALSE ("Stoped?")) -> ()
          }
          frame "unpause" {
            n152 = local write "PLL is ON ?"(TRUE ("Stoped?")) -> ()
          }
        }
      }
    }
  }
  "PLL is ON ?" <- w3
